vi "Read.vi"(8 "error in (no error)":errorcluster, 11 "StringLen_I32 in":refnum<class "StringLen_I32.lvclass">) -> (0 "error out":errorcluster, 2 "Value":T1, 3 "StringLen_I32 out":refnum<class "StringLen_I32.lvclass">)   [LabVIEW 2021, in "StringLen_I32.lvclass"]
uses:
  StringLen_I32.lvclass
  Abs_Types/I32 Integer/Support/Type.ctl
  StringLen_I32.lvclass/StringLen_I32.ctl
  Abs_Types/String/Abs_String.lvclass
  Abs_Types/I32 Integer/Abs_I32 Integer.lvclass
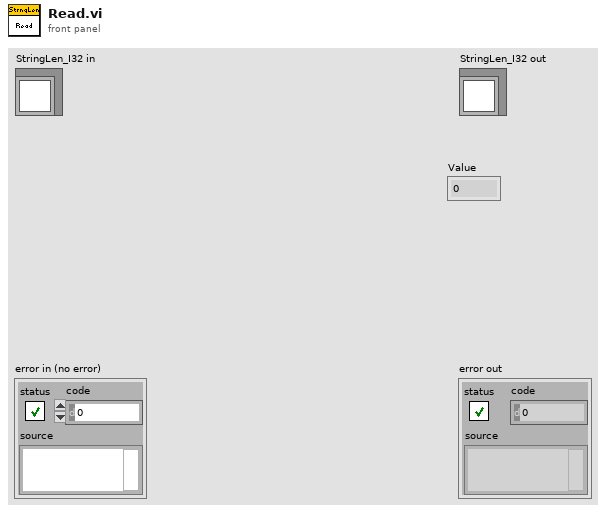
[diagram p1: front panel]
types:
  T1 = typedef "Abs_I32 Integer.lvclass/Type.ctl" = i32
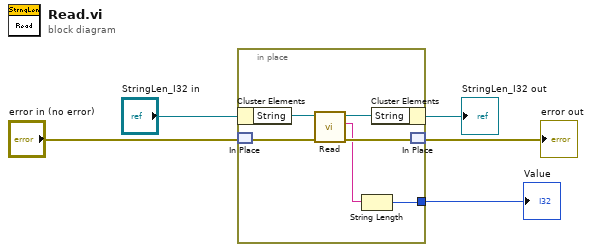
[diagram p0: block diagram]
diagram:
  n1 = in-place {
    in-place-border: [w7] -> w1
    n2 = in-place-cluster #1("StringLen_I32 in") -> ("String"=w11:refnum<class "Abs_String.lvclass">)
    n3 = in-place-match #2("error in (no error)") -> (w9:errorcluster)
    n4 = call-dynamic "Read.vi"("error in (no error)"=w9, "Abs_String in"=w11) -> ("error out"=w8:errorcluster, "String"=w6:string, "Abs_String out"=w10:refnum<class "Abs_String.lvclass">)  [unwired: 7 in]
    n5 = String Length(string=w6) -> (length=w7:i32)
    n6 = in-place-cluster #1("String"=w10) -> (→"StringLen_I32 out":refnum<class "StringLen_I32.lvclass">)
    n7 = in-place-match #2(w8) -> (→"error out":errorcluster)
  }
  "Value" <- w1
